vi "Create Structure.vi"(5 "Dims":u64[](array[numeric]), 6 "error in (no error)":errorcluster, 8 "variant":variant, 9 "Refnum in":T1) -> (0 "error out":errorcluster, 3 "Refnum out":T1)   [LabVIEW 2019]
uses:
  <vilib>/UPVI/lvhdf5/library.llb/HDF5 Ref.ctl
  <vilib>/Utility/Data Type/Type Definitions/Data Type.ctl
  <vilib>/Utility/Data Type/NI_Data Type.lvlib
panel:
  out "Fieldnames":string[](array[string])
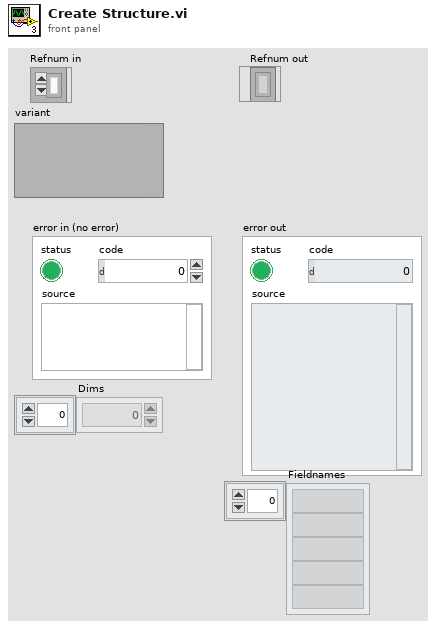
[diagram p1: front panel]
types:
  T1 = typedef "HDF5 Ref.ctl" = refnum<k1>
  T2 = typedef "NI_Data Type.lvlib/Data Type.ctl" = enum8{"Invalid Type", "Void", "I8", "I16", "I32", "I64", "U8", "U16", "U32", "U64", "Single Float", "Double Float", "Extended Float", "Single Complex", "Double Complex", "Extended Complex", "Enum U8", "Enum U16", "Enum U32", "Enum U64", "Single Float With Unit", "Double Float With Unit", "Extended Float With Unit", "Single Complex with Unit", "Double Complex with Unit", "Extended Complex with Unit", "Boolean", "String", "Path", "Picture", "Tag", "Array", "Cluster", "Variant", "LV Variant", "Waveform", "Timestamp", "Digital Waveform", "Digital Data", "ExpressData", "Refnum", "External Data", "VI", "Poly VI", "LabVIEW Class Instance", "Fixed Point", "Set Collection", "Map Collection"}
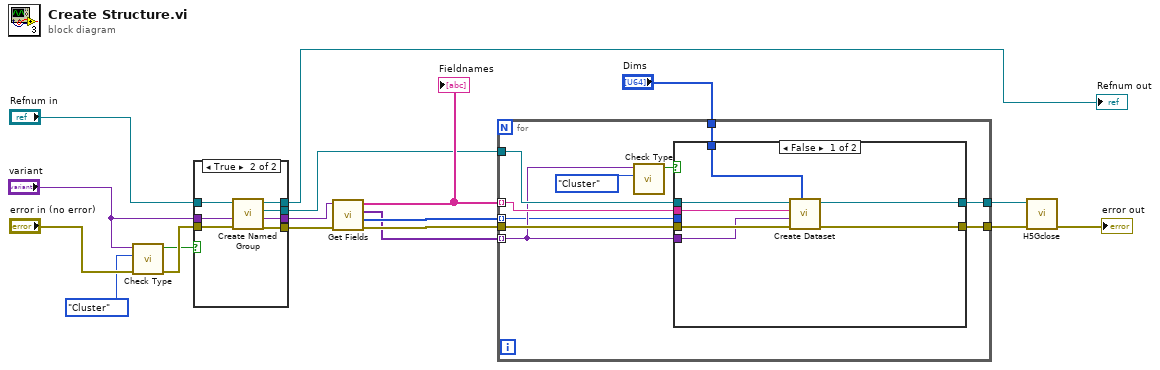
[diagram p0: block diagram]
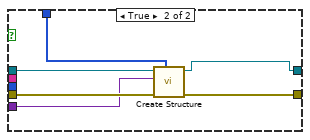
[diagram p3: hidden frame]
diagram:
  n1 = call "Check Type.vi"("error in (no error)"="error in (no error)", "type"=Data_Type."Cluster", "variant"="variant") -> ("error out"=w4:errorcluster, "is type"=w2:bool)  [unwired: 7 in]
  n2 = case shown="True" w2 {
    tunnel: w4 -> [w21 w28]
    tunnel: [w21 w27] -> w12
    tunnel: "variant" -> [w19 w26]
    tunnel: [w20 w25] -> w11
    tunnel: "Refnum in" -> [w20 w24]
    tunnel: [w20 w23] -> w9
    tunnel: [w19 w22] -> w5
    frame False {
    }
    frame True {
      n3 = call "Create Named Group.vi"("HDF5 Ref"=w24, "variant"=w26, "error in (no error)"=w28) -> ("HDF5 Ref out"=w23:T1, "HDF5 Group Ref"=w25:T1, "variant out"=w22:variant, "error out"=w27:errorcluster)  [unwired: 2 in]
    }
  }
  "Refnum out" <- w9
  n4 = call "Get Fields.vi"("error in (no error)"=w12, "variant"=w5) -> ("error out"=w18:errorcluster, "Types"=w16:T2[], "element variant array"=w15:variant[], "Fieldnames"=w17:string[])  [unwired: 5 in, 1 out]
  "Fieldnames" <- w17
  n5 = for {
    tunnel: w11 -> [w38]
    tunnel: [w37] -> w6
    tunnel: [w36] -> w8
    tunnel: w17 -> [w34] mode=indexing
    tunnel: w15 -> [w32] mode=indexing
    tunnel: w18 -> [w33]
    tunnel: w16 -> [w31] mode=indexing
    tunnel: "Dims" -> [w30]
    n6 = call "Check Type.vi"("type"=Data_Type."Cluster", "variant"=w32) -> ("is type"=w35:bool)  [unwired: 8 in, 1 out]
    n7 = case shown="False" w35 {
      tunnel: w38 -> [w45 w50]
      tunnel: w34 -> [w44 _]
      tunnel: w32 -> [w42 w48]
      tunnel: [w40 w47] -> w37
      tunnel: [w41 w49] -> w36
      tunnel: w33 -> [w43 w51]
      tunnel: w31 -> [_ _]
      tunnel: w30 -> [w39 w46]
      frame False {
        n8 = call "Create Dataset.vi"("Dims meas"=w39, "error in (no error)"=w43, "Variant"=w42, "Label.Text"=w44, "Refnum in"=w45) -> ("error out"=w41:errorcluster, "Refnum out"=w40:T1)  [unwired: 5 in]
      }
      frame True {
        n9 = call "Create Structure.vi"("Dims"=w46, "error in (no error)"=w51, "variant"=w48, "Refnum in"=w50) -> ("error out"=w49:errorcluster, "Refnum out"=w47:T1)  [unwired: 4 in]
      }
    }
  }
  n10 = call <vilib>:"H5Gclose.vi"("error in (no error)"=w8, "HDF5 Group Ref"=w6) -> ("error out"=→"error out":errorcluster)  [unwired: 7 in]
